vi "Helmholtz2D_FEM_Delaunay_Intersect.vi"(8 "Triangle":i32[](array[numeric]), 9 "Index":i32[](array[numeric]), 10 "Y":dbl[](array[numeric]), 11 "X":dbl[](array[numeric])) -> (3 "intersect?":bool)   [LabVIEW 2017, in "NI_PDE.lvlib"]
uses:
  <vilib>/gmath/NI_PDE.lvlib
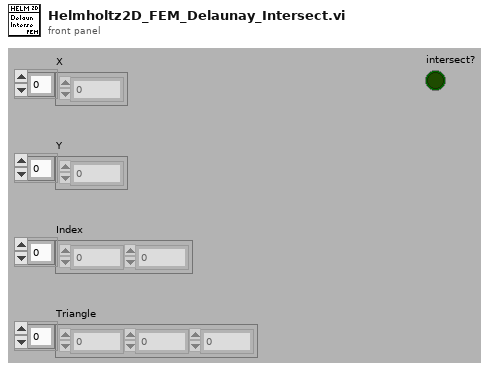
[diagram p1: front panel]
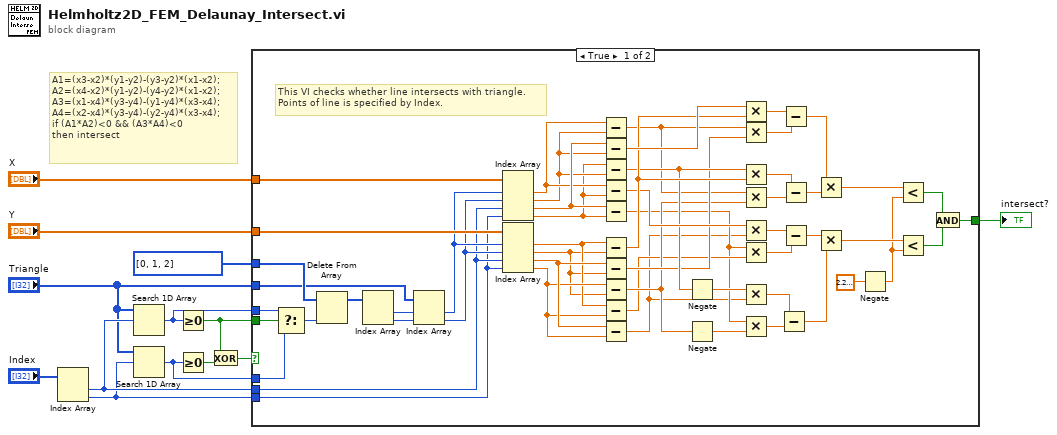
[diagram p0: block diagram]
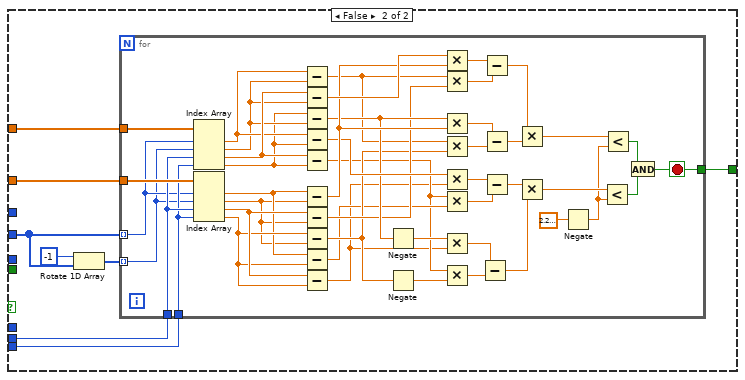
[diagram p2: hidden frame]
diagram:
  # "A1=(x3-x2)*(y1-y2)-(y3-y2)*(x1-x2);\nA2=(x4-x2)*(y1-y2)-(y4-y2)*(x1-x2);\nA3=(x1-x4)*(y3-y4)-(y1-y4)*(x3-x4);\nA4=(x2-x4)*(y3-y4)-(y2-y4)*(x3-x4);\nif (A1*A2)<0 && (A3*A4)<0\nthen intersect"
  n1 = Index Array(array="Index") -> (element #1=w7:i32, element #2=w6:i32)  [unwired: 2 in]
  n2 = Search 1D Array(1D array="Triangle", element=w7) -> (index of element=w11:i32)  [unwired: 1 out]
  n3 = Search 1D Array(1D array="Triangle", element=w6) -> (index of element=w10:i32)  [unwired: 1 out]
  n4 = Greater Or Equal To 0?(x=w11) -> (x >= 0?=w9:bool)
  n5 = Greater Or Equal To 0?(x=w10) -> (x >= 0?=w13:bool)
  n6 = Exclusive Or(1:w13, 2:w9) -> (0:w12:bool)
  n7 = case shown="True" w12 {
    tunnel: "Triangle" -> [w62 w70]
    tunnel: "X" -> [w58 w75]
    tunnel: "Y" -> [w57 w74]
    tunnel: w9 -> [w67 _]
    tunnel: w11 -> [w66 _]
    tunnel: w10 -> [w65 _]
    tunnel: i32[] [0, 1, 2] -> [w64 _]
    tunnel: w7 -> [w54 w73]
    tunnel: w6 -> [w53 w72]
    tunnel: [w44 w71] -> w5
    frame True {
      # "This VI checks whether line intersects with triangle.\nPoints of line is specified by Index."
      n8 = Select(t=w66, s=w67, f=w65) -> (s? t:f=w63:i32)
      n9 = Delete From Array(array=w64, index=w63) -> (array with subset deleted=w61:i32[])  [unwired: 1 in, 1 out]
      n10 = Index Array(array=w61) -> (element #1=w60:i32, element #2=w59:i32)  [unwired: 2 in]
      n11 = Index Array(array=w62, index #1=w60, index #2=w59) -> (element #1=w56:i32, element #2=w55:i32)
      n12 = Index Array(array=w58, index #1=w56, index #2=w55, index #3=w54, index #4=w53) -> (element #1=w50:dbl, element #2=w48:dbl, element #3=w52:dbl, element #4=w47:dbl)
      n13 = Index Array(array=w57, index #1=w56, index #2=w55, index #3=w54, index #4=w53) -> (element #1=w46:dbl, element #2=w45:dbl, element #3=w51:dbl, element #4=w49:dbl)
      n14 = Subtract(x=w50, y=w48) -> (x-y=w24:dbl)
      n15 = Subtract(x=w52, y=w48) -> (x-y=w43:dbl)
      n16 = Subtract(x=w47, y=w48) -> (x-y=w30:dbl)
      n17 = Subtract(x=w50, y=w47) -> (x-y=w35:dbl)
      n18 = Subtract(x=w52, y=w47) -> (x-y=w21:dbl)
      n19 = Subtract(x=w46, y=w45) -> (x-y=w39:dbl)
      n20 = Subtract(x=w51, y=w45) -> (x-y=w25:dbl)
      n21 = Subtract(x=w49, y=w45) -> (x-y=w23:dbl)
      n22 = Subtract(x=w46, y=w49) -> (x-y=w22:dbl)
      n23 = Subtract(x=w51, y=w49) -> (x-y=w20:dbl)
      n24 = Negate(x=w30) -> (-x=w29:dbl)
      n25 = Negate(x=w23) -> (-x=w31:dbl)
      n26 = Multiply(x=w43, y=w39) -> (x*y=w42:dbl)
      n27 = Multiply(x=w24, y=w25) -> (x*y=w41:dbl)
      n28 = Multiply(x=w30, y=w39) -> (x*y=w38:dbl)
      n29 = Multiply(x=w24, y=w23) -> (x*y=w37:dbl)
      n30 = Multiply(x=w35, y=w20) -> (x*y=w34:dbl)
      n31 = Multiply(x=w21, y=w22) -> (x*y=w33:dbl)
      n32 = Multiply(x=w29, y=w20) -> (x*y=w28:dbl)
      n33 = Multiply(x=w21, y=w31) -> (x*y=w27:dbl)
      n34 = Subtract(x=w28, y=w27) -> (x-y=w26:dbl)
      n35 = Subtract(x=w42, y=w41) -> (x-y=w40:dbl)
      n36 = Subtract(x=w38, y=w37) -> (x-y=w36:dbl)
      n37 = Subtract(x=w34, y=w33) -> (x-y=w32:dbl)
      n38 = Multiply(x=w40, y=w36) -> (x*y=w19:dbl)
      n39 = Multiply(x=w32, y=w26) -> (x*y=w16:dbl)
      n40 = Negate(x=2.220446049250313e-16) -> (-x=w14:dbl)
      n41 = Less?(x=w19, y=w14) -> (x < y?=w18:bool)
      n42 = Less?(x=w16, y=w14) -> (x < y?=w15:bool)
      n43 = And(x=w18, y=w15) -> (x .and. y?=w44:bool)
    }
    frame False {
      n44 = Rotate 1D Array(1:w70, 2:-1 ("n")) -> (0:w68:i32[])
      n45 = for {
        tunnel: w75 -> [w120]
        tunnel: w74 -> [w119]
        tunnel: w73 -> [w118]
        tunnel: w72 -> [w117]
        tunnel: [w82] -> w71
        tunnel: w70 -> [w84] mode=indexing
        tunnel: w68 -> [w83] mode=indexing
        stop <- w82 stop-if-true
        n46 = Index Array(array=w120, index #1=w84, index #2=w83, index #3=w118, index #4=w117) -> (element #1=w114:dbl, element #2=w112:dbl, element #3=w116:dbl, element #4=w111:dbl)
        n47 = Index Array(array=w119, index #1=w84, index #2=w83, index #3=w118, index #4=w117) -> (element #1=w110:dbl, element #2=w109:dbl, element #3=w115:dbl, element #4=w113:dbl)
        n48 = Subtract(x=w114, y=w112) -> (x-y=w89:dbl)
        n49 = Subtract(x=w116, y=w112) -> (x-y=w108:dbl)
        n50 = Subtract(x=w111, y=w112) -> (x-y=w95:dbl)
        n51 = Subtract(x=w114, y=w111) -> (x-y=w100:dbl)
        n52 = Subtract(x=w116, y=w111) -> (x-y=w86:dbl)
        n53 = Subtract(x=w110, y=w109) -> (x-y=w104:dbl)
        n54 = Subtract(x=w115, y=w109) -> (x-y=w90:dbl)
        n55 = Subtract(x=w113, y=w109) -> (x-y=w88:dbl)
        n56 = Subtract(x=w110, y=w113) -> (x-y=w87:dbl)
        n57 = Subtract(x=w115, y=w113) -> (x-y=w85:dbl)
        n58 = Negate(x=w95) -> (-x=w94:dbl)
        n59 = Negate(x=w88) -> (-x=w96:dbl)
        n60 = Multiply(x=w108, y=w104) -> (x*y=w107:dbl)
        n61 = Multiply(x=w89, y=w90) -> (x*y=w106:dbl)
        n62 = Multiply(x=w95, y=w104) -> (x*y=w103:dbl)
        n63 = Multiply(x=w89, y=w88) -> (x*y=w102:dbl)
        n64 = Multiply(x=w100, y=w85) -> (x*y=w99:dbl)
        n65 = Multiply(x=w86, y=w87) -> (x*y=w98:dbl)
        n66 = Multiply(x=w94, y=w85) -> (x*y=w93:dbl)
        n67 = Multiply(x=w86, y=w96) -> (x*y=w92:dbl)
        n68 = Subtract(x=w93, y=w92) -> (x-y=w91:dbl)
        n69 = Subtract(x=w107, y=w106) -> (x-y=w105:dbl)
        n70 = Subtract(x=w103, y=w102) -> (x-y=w101:dbl)
        n71 = Subtract(x=w99, y=w98) -> (x-y=w97:dbl)
        n72 = Multiply(x=w105, y=w101) -> (x*y=w80:dbl)
        n73 = Multiply(x=w97, y=w91) -> (x*y=w78:dbl)
        n74 = Negate(x=2.220446049250313e-16) -> (-x=w77:dbl)
        n75 = Less?(x=w78, y=w77) -> (x < y?=w76:bool)
        n76 = Less?(x=w80, y=w77) -> (x < y?=w79:bool)
        n77 = And(x=w79, y=w76) -> (x .and. y?=w82:bool)
      }
    }
  }
  "intersect?" <- w5
